vi "Autonomous Independent.vi"   [LabVIEW 2016]
doc: "This VI is called when autonomous begins, and will automatically be terminated when autonomous ends. You can carry out timed or sensor driven robot movement independently without needing to return to the caller."
uses:
  <vilib>/Rock Robotics/WPI/RobotDrive/WPI_RobotDriveArcadeDrive_Standard(NoSaturation).vi
  <vilib>/Rock Robotics/Network Tables/NT Write Numeric Array.vi
  <vilib>/Rock Robotics/WPI/Solenoid/WPI_SolenoidSetEnum.vi
  <vilib>/Rock Robotics/WPI/Solenoid/WPI_SolenoidValue.ctl
  <vilib>/Rock Robotics/Network Tables/NT Read String.vi
panel:
  # "Be sure to right-click and choose Data Operations>>Make Current Value default if you want to save the array values with the VI"
types:
  T1 = typedef "WPI_JoystickDevRef.ctl" = cluster{"Device":T2}
  T2 = typedef "WPI_JoystickDeviceEnum.ctl" = enum16{"USB 0", "USB 1", "USB 2", "USB 3", "USB 4", "USB 5"}
  T3 = typedef "WPI_SolenoidValue.ctl" = enum16{"Off", "On", "Forward", "Reverse"}
  T4 = typedef "WPI_SolenoidDevRef.ctl" = cluster{"DevStatus":errorcluster, "Pneumatics Control Module":u8, "Forward Solenoid Channel":T5, "Reverse Solenoid Channel":T5}
  T5 = typedef "WPI_SolenoidChannel.ctl" = enum8{"Solenoid 0", "Solenoid 1", "Solenoid 2", "Solenoid 3", "Solenoid 4", "Solenoid 5", "Solenoid 6", "Solenoid 7", "Invalid"}
  T6 = typedef "WPI_EncoderDevRef.ctl" = cluster{"DevStatus":errorcluster, "EncoderIndex":T7, "CounterIndex":T8, "DistancePerCount":dbl, "Decoding Type":T9}
  T7 = typedef "FPGA_EncoderIdx.ctl" = enum8{"Enc 0", "Enc 1", "Enc 2", "Enc 3", "Enc 4", "Enc 5", "Enc 6", "Enc 7", "Invalid"}
  T8 = typedef "FPGA_CounterCtrSystemIndex.ctl" = enum8{"Ctr 0", "Ctr 1", "Ctr 2", "Ctr 3", "Ctr 4", "Ctr 5", "Ctr 6", "Ctr 7", "Invalid"}
  T9 = typedef "WPI_EncoderType.ctl" = enum16{"1x", "2x", "4x"}
  T10 = typedef "WPI_RobotDriveDevRef.ctl" = cluster{"DevStatus":errorcluster, "Motors[]":T11[], "Square Inputs":bool, "Max Output":dbl}
  T11 = typedef "WPI_MotorControlDeviceRef.ctl" = cluster{"DeviceStatus":errorcluster, "Type":T12, "PWM":cluster{"PWM Channel":T13, "DeadBand":T14}, "CAN":cluster{"Device Number":u8, "SetOutput VI Ref":variant, "GetOutput VI Ref":variant, "Enable VI Ref":variant, "Disable VI Ref":variant, "Data":variant}, "Invert":bool}
  T12 = typedef "WPI_MotorControlType.ctl" = enum16{"PWM", "CAN"}
  T13 = typedef "FPGA_DIOPWMChannel.ctl" = enum8{"PWM 0", "PWM 1", "PWM 2", "PWM 3", "PWM 4", "PWM 5", "PWM 6", "PWM 7", "PWM 8", "PWM 9", "PWM MXP 0", "PWM MXP 1", "PWM MXP 2", "PWM MXP 3", "PWM MXP 4", "PWM MXP 5", "PWM MXP 6", "PWM MXP 7", "PWM MXP 8", "PWM MXP 9", "Invalid"}
  T14 = typedef "WPI_PWMDeadband.ctl" = cluster{"Name":string, "maxPositivePwm":i32, "minPositivePwm":i32, "centerPwm":i32, "maxNegativePwm":i32, "minNegativePwm":i32, "angularRange":u16}
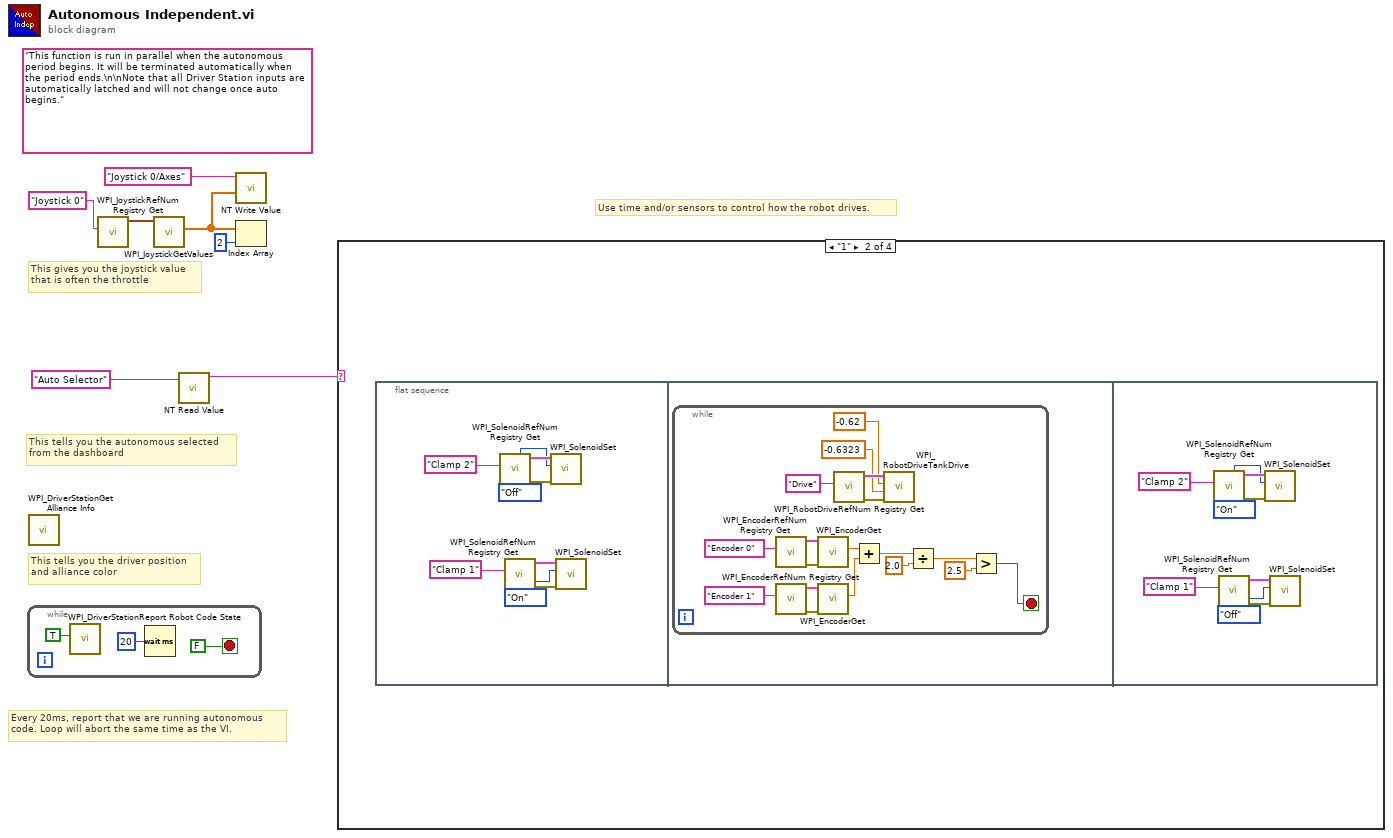
[diagram p0: block diagram]
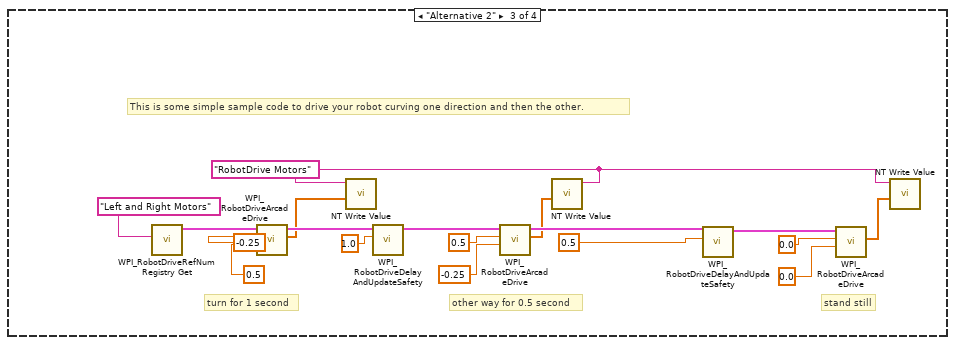
[diagram p3: hidden frame]
diagram:
  (unwired) "This function is run in parallel when the autonomous period begins. It will be terminated automatically when the period ends.\n\nNote that all Driver Station inputs are automatically latched and will not change once auto begins."
  # "This tells you the autonomous selected\nfrom the dashboard"
  # "Every 20ms, report that we are running autonomous\ncode. Loop will abort the same time as the VI."
  # "This gives you the joystick value\nthat is often the throttle"
  # "Use time and/or sensors to control how the robot drives."
  # "This tells you the driver position\nand alliance color"
  n1 = while {
    stop <- FALSE stop-if-true
    n2 = call <vilib>:"WPI_DriverStationReport Robot Code State.vi"("Autonomous"=TRUE) -> ()  [unwired: 10 in, 1 out]
    n3 = Wait (ms)(milliseconds to wait=u32 20) -> ()  [unwired: 1 out]
  }
  n4 = call <vilib>:"WPI_DriverStationGet Alliance Info.vi"() -> ()  [unwired: 12 out]
  n5 = call <vilib>:"WPI_JoystickRefNum Registry Get.vi"("refnum name"="Joystick 0") -> ("JoystickDevRef"=w6:T1)  [unwired: 1 in, 9 out]
  n6 = call <vilib>:"WPI_JoystickGetValues.vi"("JoystickDevRef"=w6) -> ("Axes"=w2:dbl[])  [unwired: 6 in, 4 out]
  n7 = call-poly <vilib>:"NT Read Value.vi"("Name"="Auto Selector") -> ("String"=w3:string)  [unwired: 9 in, 1 out]
  n8 = call-poly <vilib>:"NT Write Value.vi"("Numeric Array"=w2, "Name"="Joystick 0/Axes") -> ()  [unwired: 9 in, 1 out]
  n9 = Index Array(array=w2, index=2) -> ()  [unwired: 1 out]
  n10 = case shown="\"1\"" w3 {
    frame Default {
      # "You can put your main auto here, or you can right-click on the case and make any\nother frame be the default case."
      # "This is the frame that will execute if no selection is made, or if it is not recognized"
    }
    frame "1" {
      n11 = flat-sequence {
        frame #0 {
          n12 = call <vilib>:"WPI_SolenoidRefNum Registry Get.vi"("refnum name"="Clamp 2") -> ("error out"=w18:errorcluster, "SolenoidDevRef"=w17:T4)  [unwired: 9 in]
          n13 = call <vilib>:"WPI_SolenoidRefNum Registry Get.vi"("refnum name"="Clamp 1") -> ("error out"=w14:errorcluster, "SolenoidDevRef"=w13:T4)  [unwired: 9 in]
          n14 = call-poly <vilib>:"WPI_SolenoidSet.vi"("error in (no error)"=w18, "Value"=WPI_SolenoidValue."Off", "SolenoidDevRef"=w17) -> ()  [unwired: 7 in, 2 out]
          n15 = call-poly <vilib>:"WPI_SolenoidSet.vi"("error in (no error)"=w14, "Value"=WPI_SolenoidValue."On", "SolenoidDevRef"=w13) -> ()  [unwired: 7 in, 2 out]
        }
        frame #1 {
          n16 = while {
            stop <- w20 stop-if-true
            n17 = call <vilib>:"WPI_EncoderRefNum Registry Get.vi"("refnum name"="Encoder 0") -> ("error out"=w31:errorcluster, "EncoderDevRef"=w30:T6)  [unwired: 9 in]
            n18 = call <vilib>:"WPI_EncoderRefNum Registry Get.vi"("refnum name"="Encoder 1") -> ("error out"=w28:errorcluster, "EncoderDevRef"=w27:T6)  [unwired: 9 in]
            n19 = call <vilib>:"WPI_EncoderGet.vi"("error in (no error)"=w31, "EncoderDevRef"=w30) -> ("Distance"=w24:dbl)  [unwired: 4 in, 5 out]
            n20 = call <vilib>:"WPI_EncoderGet.vi"("error in (no error)"=w28, "EncoderDevRef"=w27) -> ("Distance"=w25:dbl)  [unwired: 4 in, 5 out]
            n21 = call <vilib>:"WPI_RobotDriveRefNum Registry Get.vi"("refnum name"="Drive") -> ("error out"=w35:errorcluster, "RobotDriveDevRef"=w36:T10)  [unwired: 9 in]
            n22 = Add(x=w24, y=w25) -> (x+y=w23:dbl)
            n23 = call <vilib>:"WPI_RobotDriveTankDrive.vi"("error in (no error)"=w35, "Right axis value"=-0.6323, "Left axis value"=-0.62, "RobotDriveDevRef"=w36) -> ()  [unwired: 5 in, 3 out]
            n24 = Divide(x=w23, y=2.0) -> (x/y=w21:dbl)
            n25 = Greater?(x=w21, y=2.5) -> (0:w20:bool)
          }
        }
        frame #2 {
          n26 = call <vilib>:"WPI_SolenoidRefNum Registry Get.vi"("refnum name"="Clamp 2") -> ("error out"=w44:errorcluster, "SolenoidDevRef"=w43:T4)  [unwired: 9 in]
          n27 = call <vilib>:"WPI_SolenoidRefNum Registry Get.vi"("refnum name"="Clamp 1") -> ("error out"=w40:errorcluster, "SolenoidDevRef"=w39:T4)  [unwired: 9 in]
          n28 = call-poly <vilib>:"WPI_SolenoidSet.vi"("error in (no error)"=w44, "Value"=WPI_SolenoidValue."On", "SolenoidDevRef"=w43) -> ()  [unwired: 7 in, 2 out]
          n29 = call-poly <vilib>:"WPI_SolenoidSet.vi"("error in (no error)"=w40, "Value"=WPI_SolenoidValue."Off", "SolenoidDevRef"=w39) -> ()  [unwired: 7 in, 2 out]
        }
      }
    }
    frame "Alternative 2" {
      w46 = "RobotDrive Motors" ("Name")
      # "This is some simple sample code to drive your robot curving one direction and then the other."
      # "stand still"
      # "other way for 0.5 second"
      # "turn for 1 second"
      n30 = call <vilib>:"WPI_RobotDriveRefNum Registry Get.vi"("refnum name"="Left and Right Motors") -> ("RobotDriveDevRef"=w62:T10)  [unwired: 1 in, 9 out]
      n31 = call-poly <vilib>:"WPI_RobotDriveArcadeDrive.vi"("Y axis value"=0.5 ("X axis value"), "X axis value"=-0.25, "RobotDriveDevRef"=w62) -> ("Motor Values"=w45:dbl[], "RobotDriveDevRef"=w55:T10)  [unwired: 1 in, 6 out]
      n32 = call-poly <vilib>:"NT Write Value.vi"("Numeric Array"=w45, "Name"=w46) -> ()  [unwired: 9 in, 1 out]
      n33 = call <vilib>:"WPI_RobotDriveDelayAndUpdateSafety.vi"("Delay (s)"=1.0, "RobotDriveDevRef"=w55) -> ("RobotDriveDevRef 2"=w56:T10)  [unwired: 8 in, 1 out]
      n34 = call-poly <vilib>:"WPI_RobotDriveArcadeDrive.vi"("Y axis value"=-0.25 ("X axis value"), "X axis value"=0.5, "RobotDriveDevRef"=w56) -> ("Motor Values"=w47:dbl[], "RobotDriveDevRef"=w57:T10)  [unwired: 1 in, 6 out]
      n35 = call-poly <vilib>:"NT Write Value.vi"("Numeric Array"=w47, "Name"=w46) -> ()  [unwired: 9 in, 1 out]
      n36 = call <vilib>:"WPI_RobotDriveDelayAndUpdateSafety.vi"("Delay (s)"=0.5, "RobotDriveDevRef"=w57) -> ("RobotDriveDevRef 2"=w58:T10)  [unwired: 8 in, 1 out]
      n37 = call-poly <vilib>:"WPI_RobotDriveArcadeDrive.vi"("Y axis value"=0.0 ("X axis value"), "X axis value"=0.0, "RobotDriveDevRef"=w58) -> ("Motor Values"=w48:dbl[])  [unwired: 1 in, 7 out]
      n38 = call-poly <vilib>:"NT Write Value.vi"("Numeric Array"=w48, "Name"=w46) -> ()  [unwired: 9 in, 1 out]
    }
    frame "Your Turn" {
    }
  }
